vi "Setup.vi"(8 "error in (no error)":errorcluster, 11 "Process Test In":refnum<class "Customer With Phone Test.lvclass">) -> (0 "error out":errorcluster, 3 "Process Test Out":refnum<class "Customer With Phone Test.lvclass">)   [LabVIEW 2020, in "Customer With Phone Test.lvclass"]
uses:
  Customer With Phone Test.lvclass
  C:/git/astemes-triarc-examples/source/Coffee Shop/Tests/Person Test/Person Test.lvclass
  Processes/People/Customers/Customer With Phone/Customer With Phone.lvclass
  C:/git/astemes-triarc-examples/source/Coffee Shop/Processes/People/Person/Person.lvclass
  Person Test/Person Test.lvclass
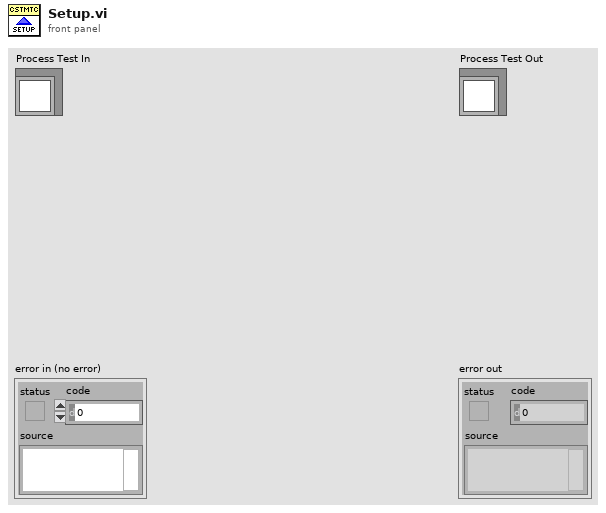
[diagram p1: front panel]
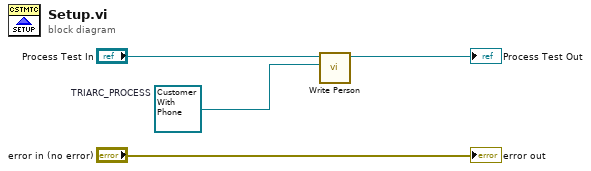
[diagram p0: block diagram]
diagram:
  w2 = refnum<class "Customer With Phone.lvclass"> refnum  # TRIARC_PROCESS
  n1 = call "Write Person.vi"("TRIARC_PROCESS"=w2, "Person Test in"="Process Test In") -> ("Person Test out"=→"Process Test Out":refnum<class "Customer With Phone Test.lvclass">)  [unwired: 9 in]
  "error out" <- "error in (no error)"
